vi "diag_output.vi"(0 "Data output file":path, 5 "Index":i32, 7 "Eventnums":i32[](array[numeric]), 9 "Polarizations":dbl[](array[numeric]), 11 "Frequency":dbl) -> ()   [LabVIEW 2015]
uses:
  <vilib>/Utility/file.llb/Write To Spreadsheet File (string).vi
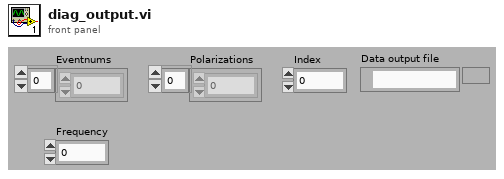
[diagram p1: front panel]
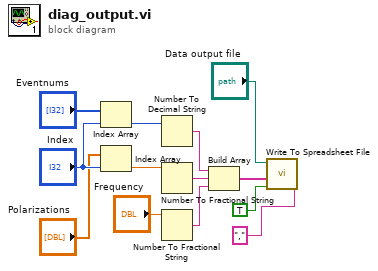
[diagram p0: block diagram]
diagram:
  n1 = Index Array(array="Eventnums", index="Index") -> (element=w4:i32)
  n2 = Index Array(array="Polarizations", index="Index") -> (element=w6:dbl)
  n3 = Number To Decimal String(number=w4) -> (decimal integer string=w12:string)  [unwired: 1 in]
  n4 = Number To Fractional String(number=w6) -> (F-format string=w3:string)  [unwired: 3 in]
  n5 = Number To Fractional String(number="Frequency") -> (F-format string=w1:string)  [unwired: 3 in]
  n6 = Build Array(w12, w3, w1) -> (w13:string[])
  n7 = call-poly <vilib>:"Write To Spreadsheet File.vi"("delimiter (\\t)"="," ("delimiter (\\t)"), "append to file? (new file:F)"=TRUE, "1D data"=w13, "file path (dialog if empty)"="Data output file") -> ()  [unwired: 4 in, 1 out]
